vi "FXP NIPLL_OnePoleARM_IIR.vi"(1 "alpha [U16.0]":fxp<+,16,0>, 3 "x":fxp<+/-,32,3>) -> (0 "y[n]":fxp<+/-,48,3>)   [LabVIEW 2012]
uses:
  <vilib>/Platform/TimedLoop/XDataNode/timing_clust.ctl
  <vilib>/Platform/TimedLoop/XDataNode/nitl_modes.ctl
  <vilib>/Platform/TimedLoop/XDataNode/wakeup.ctl
  <vilib>/rvi/Emulation/niFpgaSctlEmulationRegisterWithScheduler.vi
  <vilib>/rvi/Emulation/niFpgaSctlEmulationScheduler.vi
  <vilib>/Platform/TimedLoop/XDataNode/XDataNode.xnode
  <vilib>/rvi/FXPMathLib/FxpMul/XNode/nifxpmath_Multiplier.xnode
  <vilib>/rvi/FXPMathLib/FxpAdd/XNode/nifxpmath_Add.xnode
  <vilib>/rvi/FXPMathLib/sim/FxpSim.dll
  <vilib>/Platform/TimedLoop/XDataNode/XDNodeRunTimeDep.lvlib
panel:
  # "Pole location: 1-alpha\nH[z] = alpha/(1-z^-1 * (1-alpha))"
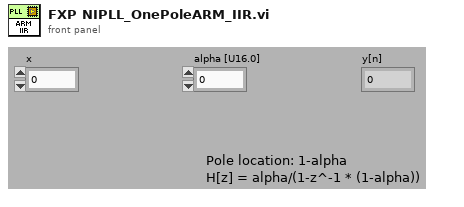
[diagram p1: front panel]
types:
  T1 = typedef "XDNodeRunTimeDep.lvlib/timing_clust.ctl" = cluster{"Expected End [f-1]":u64, "Actual End [f-1]":u64, "Finished Late? [f-1]":bool, "Expected End [i-1]":u64, "Actual End [i-1]":u64, "Finished Late? [i-1]":bool, "Expected Start [i]":u64, "Actual Start [i]":u64, "Expected Start [f]":u64, "Actual Start [f]":u64, "Source Name":string, "Structure Name":string, "Period":i64, "Deadline":i64, "Offset":i64, "Start":i64, "Priority":i32, "Timeout":i32, "Mode":T2, "Wakeup Reason":T3, "Error":errorcluster, "Source Type":string, "Secondary Source Type":string, "Global End Time":u64, "Global Start Time":u64, "Frame Duration":u64, "Iteration Duration":u64, "Assigned CPU":i32, "I/O Scan Engine Mode":u32}
  T2 = typedef "XDNodeRunTimeDep.lvlib/nitl_modes.ctl" = enum32{"No Change", "Process missed periods, maintain original phase", "Discard missed periods, maintain original phase", "Process missed periods, ignore original phase", "Discard missed periods, ignore original phase"}
  T3 = typedef "XDNodeRunTimeDep.lvlib/wakeup.ctl" = enum32{"Normal", "Aborted", "Asynchronous wakeup", "Timing source error", "Timed loop error", "Timeout"}
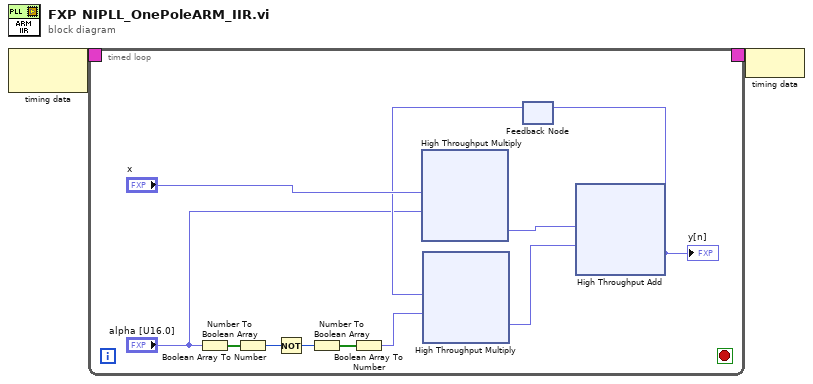
[diagram p0: block diagram]
diagram:
  n1 = node-c288() -> (w2:T1)  [unwired: 1 in]
  n2 = timed-loop {
    timing: w2 -> [_]
    timing-out: [_] -> w1
    stop <- _ stop-if-true
    n3 = Number To Boolean Array(number="alpha [U16.0]") -> (Boolean array=w8:bool[])
    n4 = Boolean Array To Number(Boolean array=w8) -> (number=w7:u16)
    n5 = Not(x=w7) -> (.not. x?=w6:u16)
    n6 = Number To Boolean Array(number=w6) -> (Boolean array=w5:bool[])
    n7 = Boolean Array To Number(Boolean array=w5) -> (number=w3:fxp<+,16,0>)
    n8 = xnode ("High Throughput Multiply")("x"="x", "y"="alpha [U16.0]") -> ("x*y"=w12:fxp<+/-,48,3>)
    n9 = feedback #1() -> (w9:fxp<+/-,48,3>)  [unwired: 1 in]
    n10 = xnode ("High Throughput Multiply")("x"=w9, "y"=w3) -> ("x*y"=w11:fxp<+/-,48,3>)
    n11 = xnode ("High Throughput Add")("x"=w12, "y"=w11) -> ("x+y"=w10:fxp<+/-,48,3>)
    "y[n]" <- w10
    n12 = feedback-in #1(w10) -> ()
  }
  n13 = node-c288(w1) -> ()
